vi "Init_Instr.vi"(8 "error in (no error)":errorcluster, 11 "EpiWrapper in":refnum<class "EpiWrapper.lvclass">) -> (0 "error out":errorcluster, 3 "EpiWrapper out":refnum<class "EpiWrapper.lvclass">)   [LabVIEW 2012, in "EpiWrapper.lvclass"]
uses:
  EpiWrapper.lvclass
  EpiWrapper.lvclass/EpiWrapper.ctl
  Instruments.lvclass
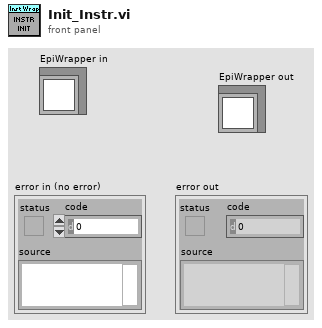
[diagram p1: front panel]
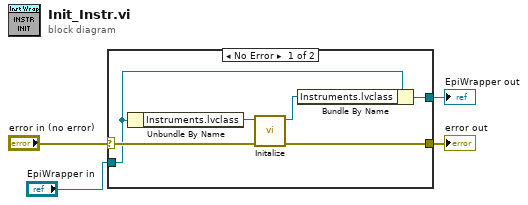
[diagram p0: block diagram]
diagram:
  n1 = case shown="No Error" "error in (no error)" {
    selector: "error in (no error)" -> [w9 w12]
    tunnel: [w8 w12] -> w3
    tunnel: [w5 w11] -> w1
    tunnel: "EpiWrapper in" -> [w7 w11]
    frame No Error {
      n2 = Unbundle By Name(w7) -> ("Instruments.lvclass"=w10:refnum<class "Instruments.lvclass">)
      n3 = call-dynamic "Initalize.vi"("error in (no error)"=w9, "Instruments in"=w10) -> ("error out"=w8:errorcluster, "Instruments out"=w6:refnum<class "Instruments.lvclass">)  [unwired: 8 in]
      n4 = Bundle By Name(cluster=w7, "Instruments.lvclass"=w6) -> (w5:refnum<class "EpiWrapper.lvclass">)
    }
    frame Error {
    }
  }
  "error out" <- w3
  "EpiWrapper out" <- w1
